vi "Proper Case (Whole String).vi"(0 "string":string, 1 "Keep Exisiting Upppercase (T)":bool=TRUE) -> (2 "proper case string":string)   [LabVIEW 2021, in "Strings.lvlib"]
uses:
  Strings.lvlib
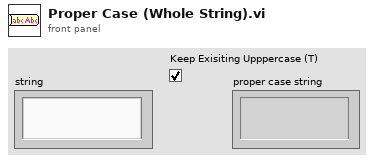
[diagram p1: front panel]
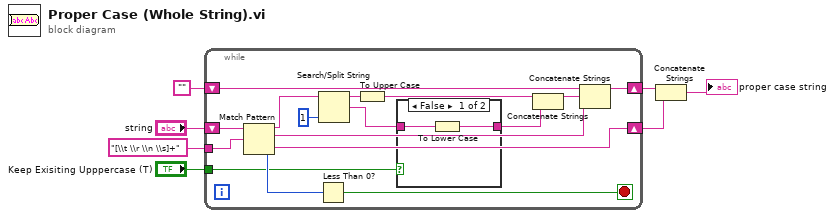
[diagram p0: block diagram]
diagram:
  n1 = while {
    shift-right: [w17] -> w2
    shift-left: "string" -> [w23]
    tunnel: "[\\t \\r \\n \\s]+" ("regular expression") -> [w22]
    shift-right: [w15] -> w4
    shift-left: "" -> [w18]
    tunnel: "Keep Exisiting Upppercase (T)" -> [w8]
    stop <- w19 stop-if-true
    n2 = Match Pattern(string=w23, regular expression=w22) -> (before substring=w21:string, match substring=w14:string, after substring=w17:string, offset past match=w20:i32)  [unwired: 1 in]
    n3 = Less Than 0?(x=w20) -> (x < 0?=w19:bool)
    n4 = Search/Split String(string=w21, offset (0)=1) -> (substring before match=w11:string, match + rest of string=w10:string)  [unwired: 1 in, 1 out]
    n5 = To Upper Case(1:w11) -> (0:w12:string)
    n6 = case shown="False" w8 {
      tunnel: [w25 w26] -> w13
      tunnel: w10 -> [w24 w26]
      frame False {
        n7 = To Lower Case(string=w24) -> (all lower case string=w25:string)
      }
      frame True {
      }
    }
    n8 = Concatenate Strings(w12, w13) -> (w16:string)
    n9 = Concatenate Strings(w18, w16, w14) -> (w15:string)
  }
  n10 = Concatenate Strings(w4, w2) -> (→"proper case string":string)
